vi "Signals.vi"() -> ()   [LabVIEW 2016]
uses:
  controls/Enum.ctl
  <vilib>/rvi/errors/niLvFpgaAdjustHostInterfaceError.vi
  SubVIs/ConvertToVoltsArray.vi
  controls/FPGAVIreferenceTypeDef.ctl
  <vilib>/rvi/interface/nirviReadWriteControl/nirviReadWriteControl.xnode
  FPGA Bitfiles/lbniAFMControlle_flexRio_controllerFPGA.lvbitx
  controls/FPGAVIreferenceTypeDefScanEngine.ctl
  FPGA Bitfiles/lbniAFMControlle_scanControl_controllerFPGAPX_N4i+37z1gG8.lvbitx
  Course Project/support/Message Queue/Message Queue.lvlib
  Course Project/support/User Event - Stop/User Event - Stop.lvlib
  NiFpgaLv.dll
panel:
  in  "channelConfiguration":enum32{"Signal"}(tab)
  in  "Signals":enum32{"Overview", "Selection"}(tab)
  in  "Analog inputs":T1={"Unit"={"Unit 1"="m", "Unit 2"="V", "Unit 3"="V", "Unit 4"="V", "Unit 5"="V", "Unit 6"="V", "Unit 7"="V", "Unit 8"="V"}, "Measurement"={"AI0 value"=0.0, "AI1 value"=0.0, "AI2 value"=0.0, "AI3 value"=-10.0, "AI4 value"=-10.0, "AI5 value"=-10.0, "AI6value"=-10.0, "AI7 value"=-10.0}, "Name"={"AI0 name"="Current", "AI1 name"="AI1", "AI2 name"="AI2", "AI3 name"="AI3", "AI4 name"="AI4", "AI5 name"="AI5", "AI6 name"="AI6", "AI7 name"="AI7"}, "Port"={"AI0"="AI0", "AI1"="AI1", "AI2"="AI2", "AI3"="AI3", "AI4"="AI4", "AI5"="AI5", "AI6"="AI6", "AI7"="AI7"}, "Calibration"={"Meas 1"=1.0, "Meas 2"=1.0, "Meas 3"=1.0, "Meas 4"=1.0, "Meas 5"=1.0, "Meas 6"=1.0, "Meas 7"=1.0, "Meas 8"=1.0}, "Offset"={"Unit 1"=0.0, "Unit 2"=0.0, "Unit 3"=0.0, "Unit 4"=0.0, "Unit 5"=0.0, "Unit 6"=0.0, "AI 106"=0.0, "Unit 8"=0.0}} {"Offset"."Unit 8" format="%#_3p"; "Offset"."AI 106" format="%#_3p"; "Offset"."Unit 6" format="%#_3p"; "Offset"."Unit 5" format="%#_3p"; "Offset"."Unit 4" format="%#_3p"; "Offset"."Unit 3" format="%#_3p"; "Offset"."Unit 2" format="%#_3p"; "Offset"."Unit 1" format="%#_3p"; "Calibration"."Meas 8" format="%#_3p"; "Calibration"."Meas 7" format="%#_3p"; "Calibration"."Meas 6" format="%#_3p"; "Calibration"."Meas 5" format="%#_3p"; "Calibration"."Meas 4" format="%#_3p"; "Calibration"."Meas 3" format="%#_3p"; "Calibration"."Meas 2" format="%#_3p"; "Calibration"."Meas 1" format="%#_3p"; "Measurement"."AI7 value" format="%#_4g"; "Measurement"."AI6value" format="%#_4g"; "Measurement"."AI5 value" format="%#_4p"; "Measurement"."AI4 value" format="%#_4p"; "Measurement"."AI3 value" format="%#_4p"; "Measurement"."AI2 value" format="%#_4p"; "Measurement"."AI1 value" format="%#_4p"; "Measurement"."AI0 value" format="%#_4p"}
  in  "Analog outputs":T2={"Unit"={"Unit 4"="V", "Unit 5"="V", "Unit 6"="V", "AI 106"="V", "Unit 8"="V"}, "Measurement"={"Meas 4"=0.0, "Meas 5"=0.0, "Meas 6"=0.0, "Meas 7"=0.0, "Meas 8"=0.0}, "Name"={"AO3 name"="AO3", "AO4 name"="Bias", "AO5 name"="DC Motor", "AO6 name"="AO6", "AO7 name"="AO7"}, "Port"={"A03"="AO3", "A04"="AO4", "A05"="AO5", "A06"="AO6", "A00"="AO7"}, "Calibration"={"Meas 4"=1.0, "Meas 5"=1.0, "Meas 6"=1.0, "Meas 7"=1.0, "Meas 8"=1.0}, "Offset"={"Unit 4"=0.0, "Unit 5"=0.0, "Unit 6"=0.0, "AI 106"=0.0, "Unit 8"=0.0}} {"Offset"."Unit 8" format="%#_3p"; "Offset"."AI 106" format="%#_3p"; "Offset"."Unit 6" format="%#_3p"; "Offset"."Unit 5" format="%#_3p"; "Offset"."Unit 4" format="%#_3p"; "Calibration"."Meas 8" format="%#_3p"; "Calibration"."Meas 7" format="%#_3p"; "Calibration"."Meas 6" format="%#_3p"; "Calibration"."Meas 5" format="%#_3p"; "Calibration"."Meas 4" format="%#_3p"; "Measurement"."Meas 8" format="%#_4p"; "Measurement"."Meas 7" format="%#_4p"; "Measurement"."Meas 6" format="%#_4p"; "Measurement"."Meas 5" format="%#_4p"; "Measurement"."Meas 4" format="%#_4p"}
  in  "XYZ":T3={"Unit"={"Unit 1"="m", "Unit 2"="m", "Unit 3"="m"}, "Measurement"={"Meas 1"=0.0, "Meas 2"=0.0, "Meas 3"=0.0}, "Name"={"AO0 name"="X", "AO1 name"="Y", "AO2 name"="Z"}, "Port"={"A00"="AO0", "A01"="AO1", "A02"="AO2"}, "Calibration"={"Meas 1"=1.0, "Meas 2"=1.0, "Meas 3"=1.0}, "Offset"={"Unit 1"=0.0, "Unit 2"=0.0, "Unit 3"=0.0}} {"Offset"."Unit 3" format="%#_3p"; "Offset"."Unit 2" format="%#_3p"; "Offset"."Unit 1" format="%#_3p"; "Calibration"."Meas 3" format="%#_3p"; "Calibration"."Meas 2" format="%#_3p"; "Calibration"."Meas 1" format="%#_3p"; "Measurement"."Meas 3" format="%#_4p"; "Measurement"."Meas 2" format="%#_4p"; "Measurement"."Meas 1" format="%#_4p"}
  in  "Save to config file":bool
  in  "Channels to save":i32[](listbox)=[0, 1, 2, 3, 4, 5, 6, 7]
  in  "Update Time":i32=500
  in  "SavingChoice":T4={"Units"=-1, "Saving"={"Fwd"=[0, 1, 3, 4, 5], "Bwd"=[0, 1]}, "x"=[]}
  in  "assignementChoice":enum32{"Selection", "Overview", "Assignment"}(radio)
  # "Ch"
  # "Name"
  # "Value"
  # "Unit"
  # "Offset"
  # "Cal"
  # "Select the channels to save.\nFor multiple selection, press ctrl + mouse."
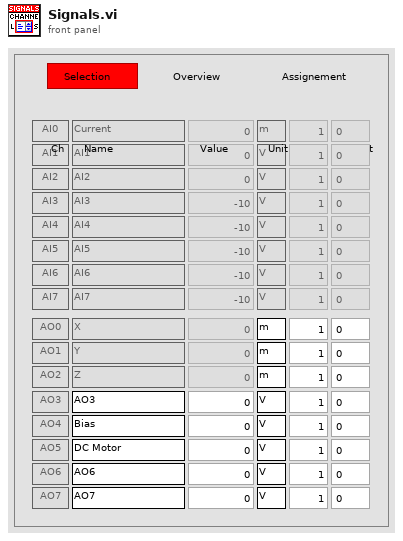
[diagram p1: front panel]
types:
  T1 = cluster{"Unit":cluster{"Unit 1":string, "Unit 2":string, "Unit 3":string, "Unit 4":string, "Unit 5":string, "Unit 6":string, "Unit 7":string, "Unit 8":string}, "Measurement":cluster{"AI0 value":dbl, "AI1 value":dbl, "AI2 value":dbl, "AI3 value":dbl, "AI4 value":dbl, "AI5 value":dbl, "AI6value":dbl, "AI7 value":dbl}, "Name":cluster{"AI0 name":string, "AI1 name":string, "AI2 name":string, "AI3 name":string, "AI4 name":string, "AI5 name":string, "AI6 name":string, "AI7 name":string}, "Port":cluster{"AI0":string, "AI1":string, "AI2":string, "AI3":string, "AI4":string, "AI5":string, "AI6":string, "AI7":string}, "Calibration":cluster{"Meas 1":dbl, "Meas 2":dbl, "Meas 3":dbl, "Meas 4":dbl, "Meas 5":dbl, "Meas 6":dbl, "Meas 7":dbl, "Meas 8":dbl}, "Offset":cluster{"Unit 1":dbl, "Unit 2":dbl, "Unit 3":dbl, "Unit 4":dbl, "Unit 5":dbl, "Unit 6":dbl, "AI 106":dbl, "Unit 8":dbl}}
  T2 = cluster{"Unit":cluster{"Unit 4":string, "Unit 5":string, "Unit 6":string, "AI 106":string, "Unit 8":string}, "Measurement":cluster{"Meas 4":dbl, "Meas 5":dbl, "Meas 6":dbl, "Meas 7":dbl, "Meas 8":dbl}, "Name":cluster{"AO3 name":string, "AO4 name":string, "AO5 name":string, "AO6 name":string, "AO7 name":string}, "Port":cluster{"A03":string, "A04":string, "A05":string, "A06":string, "A00":string}, "Calibration":cluster{"Meas 4":dbl, "Meas 5":dbl, "Meas 6":dbl, "Meas 7":dbl, "Meas 8":dbl}, "Offset":cluster{"Unit 4":dbl, "Unit 5":dbl, "Unit 6":dbl, "AI 106":dbl, "Unit 8":dbl}}
  T3 = cluster{"Unit":cluster{"Unit 1":string, "Unit 2":string, "Unit 3":string}, "Measurement":cluster{"Meas 1":dbl, "Meas 2":dbl, "Meas 3":dbl}, "Name":cluster{"AO0 name":string, "AO1 name":string, "AO2 name":string}, "Port":cluster{"A00":string, "A01":string, "A02":string}, "Calibration":cluster{"Meas 1":dbl, "Meas 2":dbl, "Meas 3":dbl}, "Offset":cluster{"Unit 1":dbl, "Unit 2":dbl, "Unit 3":dbl}}
  T4 = cluster{"Units":i32, "Saving":cluster{"Fwd":i32[], "Bwd":i32[]}, "x":i32[]}
  T5 = typedef "Enum.ctl" = enum16{"Init", "Read", "Write"}
  T6 = enum8{"Enabled", "Disabled", "Disabled and Grayed Out"}
  T7 = typedef "Message Queue.lvlib/All Message Queues.ctl" = cluster{"IU":refnum<queue>}
  T8 = typedef "FPGAVIreferenceTypeDef.ctl" = refnum<k20>
  T9 = typedef "FPGAVIreferenceTypeDefScanEngine.ctl" = refnum<k20>
  T10 = cluster{"Unit 1":string, "Unit 2":string, "Unit 3":string}
  T11 = cluster{"Meas 1":dbl, "Meas 2":dbl, "Meas 3":dbl}
  T12 = cluster{"Unit 1":dbl, "Unit 2":dbl, "Unit 3":dbl}
  T13 = cluster{"Unit 1":string, "Unit 2":string, "Unit 3":string, "Unit 4":string, "Unit 5":string, "Unit 6":string, "Unit 7":string, "Unit 8":string}
  T14 = cluster{"Unit 4":string, "Unit 5":string, "Unit 6":string, "AI 106":string, "Unit 8":string}
  T15 = cluster{"Unit 1":dbl, "Unit 2":dbl, "Unit 3":dbl, "Unit 4":dbl, "Unit 5":dbl, "Unit 6":dbl, "AI 106":dbl, "Unit 8":dbl}
  T16 = cluster{"Unit 4":dbl, "Unit 5":dbl, "Unit 6":dbl, "AI 106":dbl, "Unit 8":dbl}
  T17 = cluster{"Meas 1":dbl, "Meas 2":dbl, "Meas 3":dbl, "Meas 4":dbl, "Meas 5":dbl, "Meas 6":dbl, "Meas 7":dbl, "Meas 8":dbl}
  T18 = cluster{"Meas 4":dbl, "Meas 5":dbl, "Meas 6":dbl, "Meas 7":dbl, "Meas 8":dbl}
  T19 = cluster{"channelsToSaveOut":u8[], "Units":string[], "Saving":cluster{"Fwd":i32[], "Bwd":i32[]}, "x":i32[]}
  T20 = cluster{"Units":string[], "Offsets":dbl[], "Calibrations":dbl[]}
  T21 = cluster{"calibName":string[], "calibParameters":cluster{"Sensitivity":cluster{"Sens X":dbl, "Sens Y":dbl, "Sens Z":dbl}, "Range":cluster{"Range X":dbl, "Range Y":dbl, "Range Z":dbl}, "HV gain":cluster{"HV gain X":dbl, "HV gain Y":dbl, "HV gain Z":dbl}}[], "calibIndex":i32}
  T22 = cluster{"Sensitivity":cluster{"Sens X":dbl, "Sens Y":dbl, "Sens Z":dbl}, "Range":cluster{"Range X":dbl, "Range Y":dbl, "Range Z":dbl}, "HV gain":cluster{"HV gain X":dbl, "HV gain Y":dbl, "HV gain Z":dbl}}[]
  T23 = cluster{"Sensitivity":cluster{"Sens X":dbl, "Sens Y":dbl, "Sens Z":dbl}, "Range":cluster{"Range X":dbl, "Range Y":dbl, "Range Z":dbl}, "HV gain":cluster{"HV gain X":dbl, "HV gain Y":dbl, "HV gain Z":dbl}}
  T24 = cluster{"AI0 value":dbl, "AI1 value":dbl, "AI2 value":dbl, "AI3 value":dbl, "AI4 value":dbl, "AI5 value":dbl, "AI6value":dbl, "AI7 value":dbl}
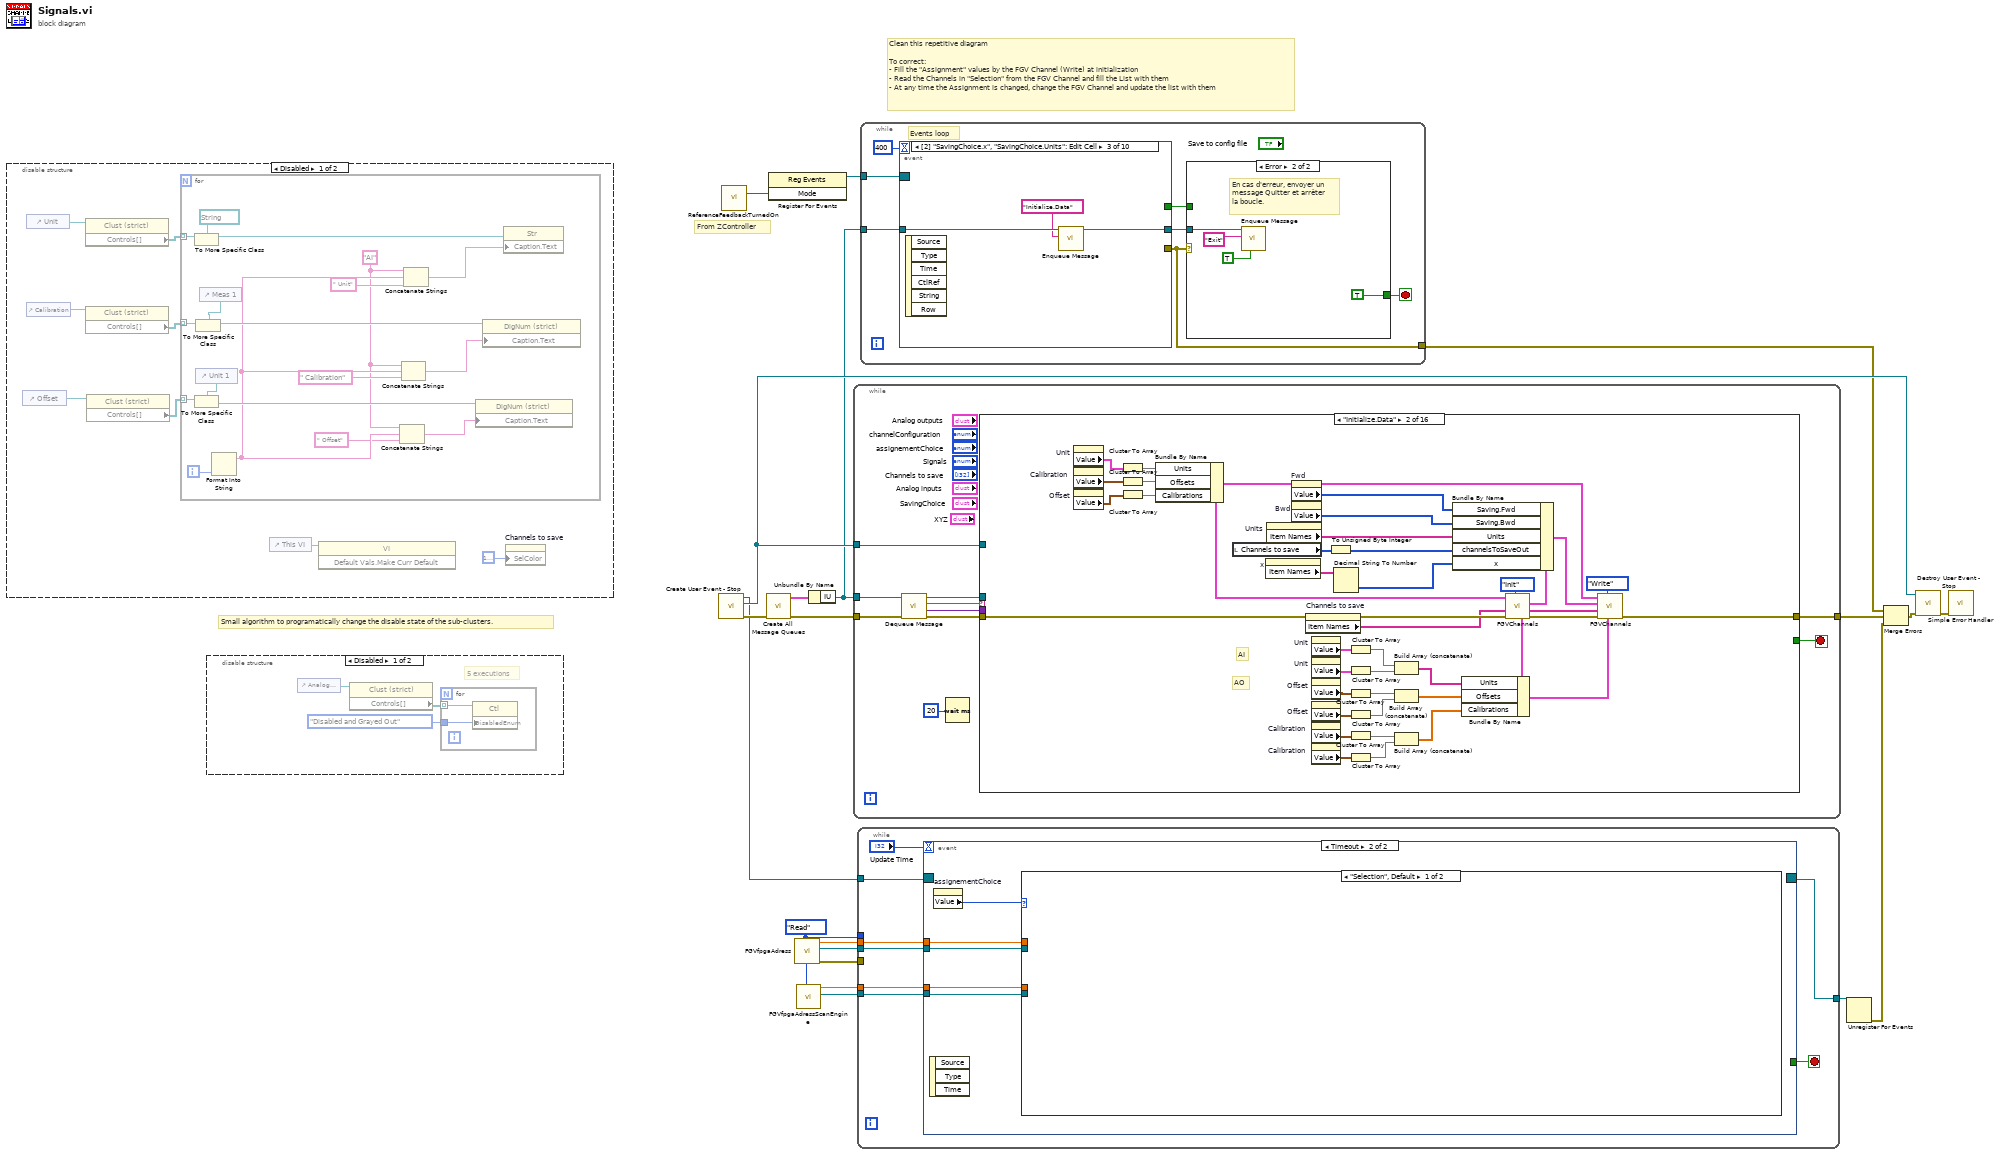
[diagram p0: block diagram]
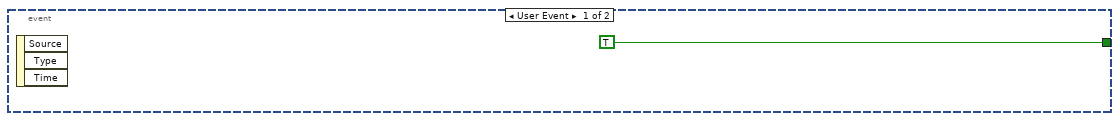
[diagram p2: hidden frame]
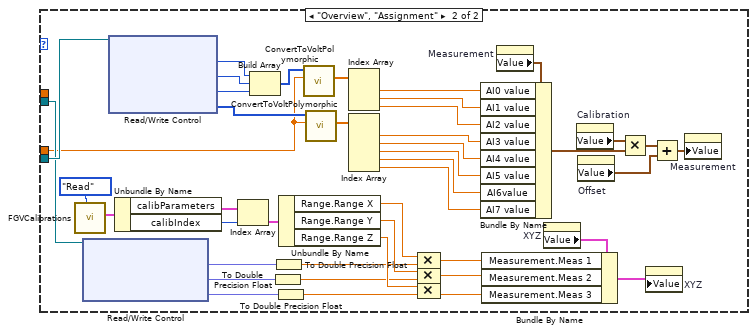
[diagram p3: hidden frame]
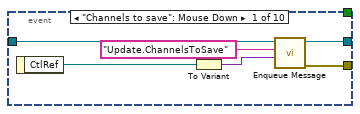
[diagram p5: hidden frame]
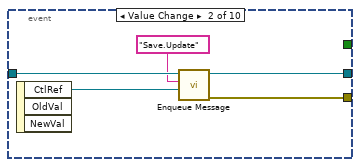
[diagram p6: hidden frame]
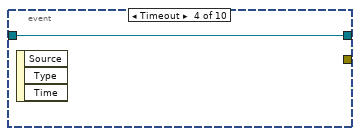
[diagram p7: hidden frame]
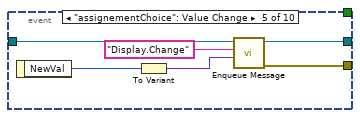
[diagram p8: hidden frame]
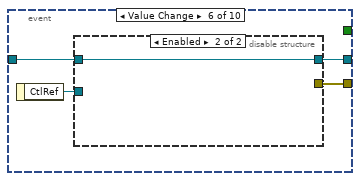
[diagram p9: hidden frame]
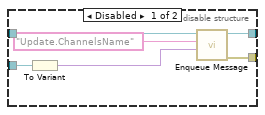
[diagram p10: hidden frame]
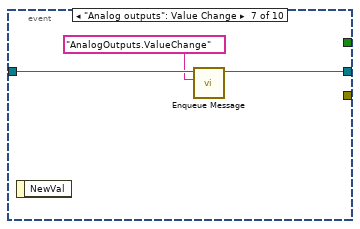
[diagram p11: hidden frame]
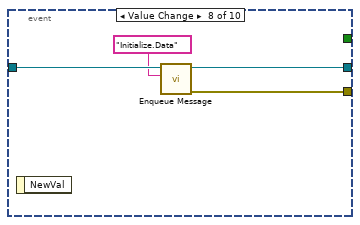
[diagram p12: hidden frame]
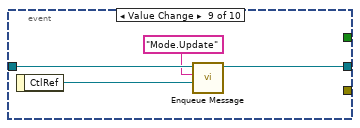
[diagram p13: hidden frame]
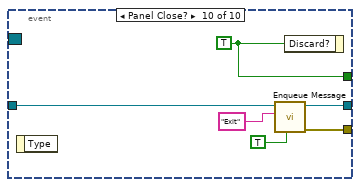
[diagram p14: hidden frame]
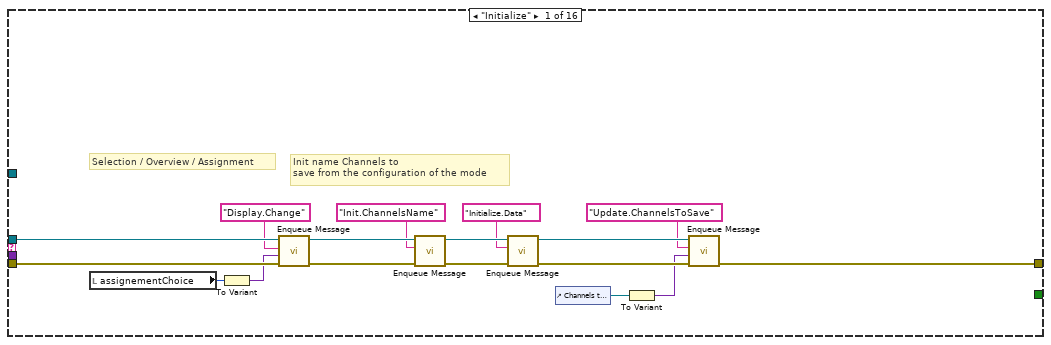
[diagram p15: hidden frame]
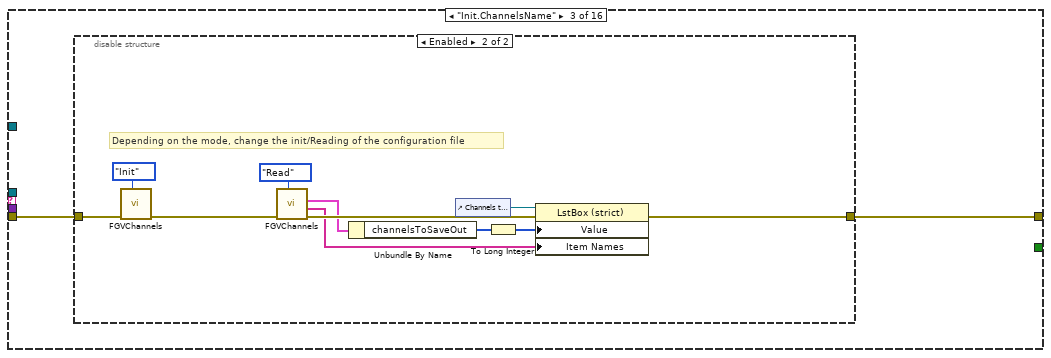
[diagram p16: hidden frame]
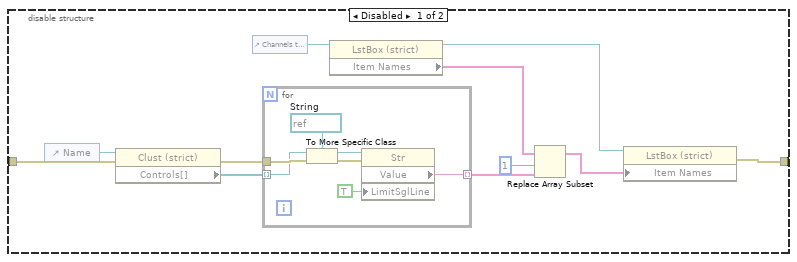
[diagram p17: hidden frame]
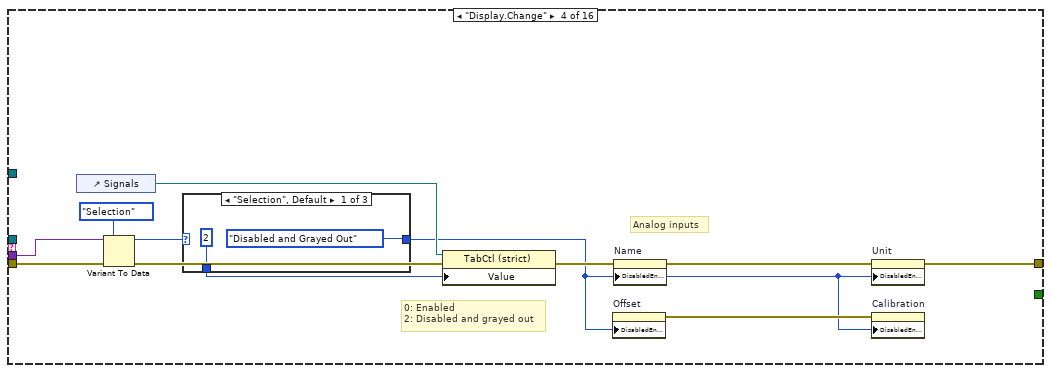
[diagram p18: hidden frame]
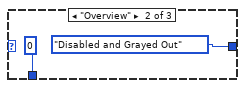
[diagram p19: hidden frame]
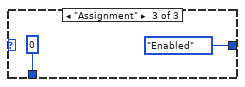
[diagram p20: hidden frame]
diagram:
  w6 = Enum."Read" ("Enum")
  # "Clean this repetitive diagram\n\nTo correct:\n- Fill the \"Assignment\" values by the FGV Channel (Write) at initialization\n- Read the Channels in \"Selection\" from the FGV Channel and fill the List with them\n- At any time the Assignment is changed, change the FGV Channel and update the list with them"
  # "From ZController"
  # "Small algorithm to programatically change the disable state of the sub-clusters."
  n1 = disable-structure shown="Disabled" {
    frame Disabled {
      n2 = control-ref of="Offset"() -> (w26:refnum<vi>)
      n3 = control-ref of="Unit"() -> (w28:refnum<vi>)
      n4 = control-ref of="Calibration"() -> (w27:refnum<vi>)
      n5 = property class="Clust (strict)"(reference=w28) -> ("Controls[]"=w25:refnum<vi>[])  [unwired: 1 in, 2 out]
      n6 = property class="Clust (strict)"(reference=w27) -> ("Controls[]"=w24:refnum<vi>[])  [unwired: 1 in, 2 out]
      n7 = property class="Clust (strict)"(reference=w26) -> ("Controls[]"=w23:refnum<vi>[])  [unwired: 1 in, 2 out]
      n8 = for {
        tunnel: w25 -> [w46] mode=indexing
        tunnel: w24 -> [w44] mode=indexing
        tunnel: w23 -> [w43] mode=indexing
        i -> [w39]
        w29 = "AI"
        n9 = To More Specific Class(target class=refnum<vi> refnum ("Unit 1"), reference=w46) -> (specific class reference=w40:refnum<vi>)  [unwired: 1 in, 1 out]
        n10 = control-ref of="Unit 1"() -> (w30:refnum<vi>)
        n11 = To More Specific Class(target class=w30, reference=w43) -> (specific class reference=w42:refnum<vi>)  [unwired: 1 in, 1 out]
        n12 = control-ref of="Meas 1"() -> (w31:refnum<vi>)
        n13 = To More Specific Class(target class=w31, reference=w44) -> (specific class reference=w41:refnum<vi>)  [unwired: 1 in, 1 out]
        n14 = Format Into String(w39) -> (resulting string=w38:string)  [unwired: 3 in, 1 out]
        n15 = Concatenate Strings(w29, w38, " Offset") -> (w32:string)
        n16 = Concatenate Strings(w29, w38, " Calibration") -> (w33:string)
        n17 = Concatenate Strings(w29, w38, " Unit") -> (w34:string)
        n18 = property class="DigNum (strict)"(reference=w42, "Caption.Text"=w32) -> ()  [unwired: 1 in, 2 out]
        n19 = property class="DigNum (strict)"(reference=w41, "Caption.Text"=w33) -> ()  [unwired: 1 in, 2 out]
        n20 = property class="Str"(reference=w40, "Caption.Text"=w34) -> ()  [unwired: 1 in, 2 out]
      }
      n21 = control-ref of="This VI"() -> (w22:refnum<vi>)
      n22 = invoke class="VI" method="Default Vals.Make Curr Default"(reference=w22) -> ()  [unwired: 2 in, 3 out]
      n23 = property on="Channels to save" class="LstBox (strict)"("SelColor"=u32 16777224) -> ()  [unwired: 2 in, 2 out]
    }
    frame Enabled {
    }
  }
  n24 = disable-structure shown="Disabled" {
    frame Disabled {
      # "5 executions"
      n25 = control-ref of="Analog inputs"() -> (w49:refnum<vi>)
      n26 = property class="Clust (strict)"(reference=w49) -> ("Controls[]"=w48:refnum<vi>[])  [unwired: 1 in, 2 out]
      n27 = for {
        tunnel: w48 -> [w51] mode=indexing
        tunnel: T6."Disabled and Grayed Out" ("Disabled") -> [w50]
        n28 = property class="Ctl"(reference=w51, "DisabledEnum"=w50) -> ()  [unwired: 1 in, 2 out]
      }
    }
    frame Enabled {
    }
  }
  n29 = call "Create User Event - Stop.vi"() -> ("sortie d'erreur"=w17:errorcluster, "Événement utilisateur - Arrêt"=w20:refnum<user-event>, "Refnum Enregistrement à l'événement Arrêt"=w10:refnum<event-registration>)  [unwired: 9 in]
  n30 = call "ReferenceFeedbackTurnedOn.vi"() -> ("Mode"=w1:refnum<vi>)  [unwired: 9 in, 2 out]
  n31 = call "Create All Message Queues.vi"("ErrorIn"=w17) -> ("ErrorOut"=w13:errorcluster, "MessageQueueOut"=w14:T7)  [unwired: 9 in]
  n32 = register-events(w1) -> (reference out=w2:refnum<event-registration>)  [unwired: 2 in, 1 out]
  n33 = call "FGVfpgaAdress.vi"("Enum"=w6) -> ("error out"=w12:errorcluster, "FPGA VI Reference Out"=w11:T8, "voltageRange(+/-)Out"=w3:dbl)  [unwired: 5 in, 3 out]
  n34 = call "FGVfpgaAdressScanEngine.vi"("Enum"=w6) -> ("FPGA.SEout"=w5:T9, "voltageRange(+/-)Out"=w4:dbl)  [unwired: 6 in, 3 out]
  n35 = Unbundle By Name(w14) -> ("IU"=w16:refnum<queue>)
  n36 = while {
    tunnel: w16 -> [w53]
    tunnel: w20 -> [w59]
    tunnel: w13 -> [w58]
    tunnel: [w60] -> w15
    stop <- w61 stop-if-true
    n37 = call "Dequeue Message.vi"("entrée d'erreur (pas d'erreur)"=w58, "File d'attente de messages"=w53) -> ("sortie d'erreur"=w57:errorcluster, "Données de message"=w55:variant, "Message"=w56:string, "File d'attente de message dup."=w54:refnum<queue>)  [unwired: 6 in]
    n38 = Wait (ms)(milliseconds to wait=u32 20) -> ()  [unwired: 1 out]
    n39 = case "Conditions des messages" shown="\"Initialize.Data\"" w56 {
      selector: w56 -> [_ _ _ _ _ _ _ _ _ _ _ _ _ _ _ w408]
      tunnel: w54 -> [w75 _ _ _ _ _ _ _ _ _ _ _ w386 w397 w404 _]
      tunnel: w57 -> [w74 w95 w119 w161 w186 w228 w255 w275 w331 w342 w366 w372 w374 w395 w400 _]
      tunnel: [w66 w116 w120 w153 w180 w194 w256 w288 w330 w338 w359 w372 w380 w394 w401 w406] -> w60
      tunnel: [_ _ _ _ _ _ _ _ _ _ _ _ _ _ TRUE _] -> w61
      tunnel: w55 -> [_ _ _ w160 w185 w227 _ _ _ _ w365 _ _ _ _ _]
      tunnel: w59 -> [_ _ _ _ _ _ _ _ _ _ _ _ _ _ w399 _]
      frame "Initialize" {
        # "Selection / Overview / Assignment"
        # "Init name Channels to \nsave from the configuration of the mode"
        n40 = local read "assignementChoice"() -> (w62:enum32{"Selection", "Overview", "Assignment"})
        n41 = To Variant(anything=w62) -> (Variant=w63:variant)
        n42 = call "Enqueue Message.vi"("error in"=w74, "Data"=w63, "Message"="Display.Change", "Queue"=w75) -> ("error out"=w71:errorcluster, "Queue dup."=w76:refnum<queue>)  [unwired: 6 in]
        n43 = call "Enqueue Message.vi"("error in"=w71, "Message"="Init.ChannelsName", "Queue"=w76) -> ("error out"=w70:errorcluster, "Queue dup."=w77:refnum<queue>)  [unwired: 7 in]
        n44 = call "Enqueue Message.vi"("error in"=w70, "Message"="Initialize.Data", "Queue"=w77) -> ("error out"=w67:errorcluster, "Queue dup."=w78:refnum<queue>)  [unwired: 7 in]
        n45 = control-ref of="Channels to save"() -> (w65:refnum<vi>)
        n46 = To Variant(anything=w65) -> (Variant=w64:variant)
        n47 = call "Enqueue Message.vi"("error in"=w67, "Data"=w64, "Message"="Update.ChannelsToSave", "Queue"=w78) -> ("error out"=w66:errorcluster)  [unwired: 6 in, 1 out]
      }
      frame "Initialize.Data" {
        # "AO"
        # "AI"
        n48 = property on="Unit" class="Clust (strict)"() -> ("Value"=w91:T10)  [unwired: 2 in, 2 out]
        n49 = property on="Calibration" class="Clust (strict)"() -> ("Value"=w89:T11)  [unwired: 2 in, 2 out]
        n50 = property on="Offset" class="Clust (strict)"() -> ("Value"=w87:T12)  [unwired: 2 in, 2 out]
        n51 = Cluster To Array(cluster=w91) -> (array=w90:string[])
        n52 = Cluster To Array(cluster=w89) -> (array=w88:dbl[])
        n53 = Cluster To Array(cluster=w87) -> (array=w86:dbl[])
        n54 = local read "Channels to save"() -> (w113:i32[])
        n55 = property on="x" class="LstBox (strict)"() -> ("Item Names"=w80:string[])  [unwired: 2 in, 2 out]
        n56 = property on="Units" class="LstBox (strict)"() -> ("Item Names"=w111:string[])  [unwired: 2 in, 2 out]
        n57 = property on="Fwd" class="LstBox (strict)"() -> ("Value"=w109:i32[])  [unwired: 2 in, 2 out]
        n58 = property on="Bwd" class="LstBox (strict)"() -> ("Value"=w110:i32[])  [unwired: 2 in, 2 out]
        n59 = property on="Channels to save" class="LstBox (strict)"(error in=w95) -> (error out=w118:errorcluster, "Item Names"=w92:string[])  [unwired: 1 in, 1 out]
        n60 = property on="Unit" class="Clust (strict)"() -> ("Value"=w85:T13)  [unwired: 2 in, 2 out]
        n61 = property on="Unit" class="Clust (strict)"() -> ("Value"=w84:T14)  [unwired: 2 in, 2 out]
        n62 = property on="Offset" class="Clust (strict)"() -> ("Value"=w104:T15)  [unwired: 2 in, 2 out]
        n63 = property on="Offset" class="Clust (strict)"() -> ("Value"=w102:T16)  [unwired: 2 in, 2 out]
        n64 = property on="Calibration" class="Clust (strict)"() -> ("Value"=w105:T17)  [unwired: 2 in, 2 out]
        n65 = property on="Calibration" class="Clust (strict)"() -> ("Value"=w103:T18)  [unwired: 2 in, 2 out]
        n66 = To Unsigned Byte Integer(number=w113) -> (unsigned 8bit integer=w112:u8[])
        n67 = Decimal String To Number(string=w80) -> (number=w79:i32[])  [unwired: 2 in, 1 out]
        n68 = Cluster To Array(cluster=w85) -> (array=w83:string[])
        n69 = Cluster To Array(cluster=w84) -> (array=w82:string[])
        n70 = Cluster To Array(cluster=w104) -> (array=w100:dbl[])
        n71 = Cluster To Array(cluster=w102) -> (array=w101:dbl[])
        n72 = Cluster To Array(cluster=w105) -> (array=w99:dbl[])
        n73 = Cluster To Array(cluster=w103) -> (array=w98:dbl[])
        n74 = Build Array (concatenate)(w83, w82) -> (w81:string[])
        n75 = Build Array (concatenate)(w100, w101) -> (w97:dbl[])
        n76 = Build Array (concatenate)(w99, w98) -> (w96:dbl[])
        n77 = call "FGVChannels.vi"("Enum"=Enum."Init") -> ("SavingChoiceOut"=w114:T19, "XYZ Units/Cal/Offset Out"=w93:T20, "Units/Cal/Offset Out"=w107:T20)  [unwired: 6 in, 2 out]
        n78 = Bundle By Name(cluster=w93, "Units"=w90, "Offsets"=w88, "Calibrations"=w86) -> (w94:T20)
        n79 = Bundle By Name(cluster=w114, "Saving.Fwd"=w109, "Saving.Bwd"=w110, "Units"=w111, "channelsToSaveOut"=w112, "x"=w79) -> (w108:T19)
        n80 = Bundle By Name(cluster=w107, "Units"=w81, "Offsets"=w97, "Calibrations"=w96) -> (w106:T20)
        n81 = call "FGVChannels.vi"("Units/Cal/Offset In"=w106, "Enum"=Enum."Write", "error in"=w118, "channelsNamesIn"=w92, "SavingChoiceIn"=w108, "XYZ Units/Cal/Offset In"=w94) -> ("error out"=w116:errorcluster)  [unwired: 1 in, 4 out]
      }
      frame "Init.ChannelsName" {
        n82 = disable-structure shown="Enabled" {
          disable-tunnel: [w125 w144] -> w120
          disable-tunnel: w119 -> [w121 w147]
          frame Disabled {
            n83 = control-ref of="Name"() -> (w122:refnum<vi>)
            n84 = property class="Clust (strict)"(reference=w122, error in=w121) -> (error out=w124:errorcluster, "Controls[]"=w123:refnum<vi>[])  [unwired: 1 out]
            n85 = control-ref of="Channels to save"() -> (w131:refnum<vi>)
            n86 = for {
              tunnel: w124 -> [w137]
              tunnel: [w134] -> w129 mode=indexing
              tunnel: w123 -> [w132] mode=indexing
              w138 = refnum<vi> refnum  # String
              n87 = To More Specific Class(target class=w138, reference=w132, error in=w137) -> (specific class reference=w136:refnum<vi>, error out=w135:errorcluster)
              n88 = property class="Str"(reference=w136, error in=w135, "LimitSglLine"=TRUE ("Limit To Single Line?")) -> ("Value"=w134:string)  [unwired: 2 out]
            }
            n89 = property class="LstBox (strict)"(reference=w131) -> (reference out=w127:refnum<vi>, "Item Names"=w130:string[])  [unwired: 1 in, 1 out]
            n90 = Replace Array Subset(array=w130, new element=w129, index=1) -> (w128:string[])
            n91 = property class="LstBox (strict)"(reference=w127, "Item Names"=w128) -> (error out=w125:errorcluster)  [unwired: 1 in, 1 out]
          }
          frame Enabled {
            # "Depending on the mode, change the init/Reading of the configuration file"
            n92 = call "FGVChannels.vi"("Enum"=Enum."Init", "error in"=w147) -> ("error out"=w146:errorcluster)  [unwired: 5 in, 4 out]
            n93 = call "FGVChannels.vi"("Enum"=Enum."Read", "error in"=w146) -> ("error out"=w145:errorcluster, "channelsNamesOut"=w142:string[], "SavingChoiceOut"=w141:T19)  [unwired: 5 in, 2 out]
            n94 = Unbundle By Name(w141) -> ("channelsToSaveOut"=w140:u8[])
            n95 = control-ref of="Channels to save"() -> (w143:refnum<vi>)
            n96 = To Long Integer(number=w140) -> (32bit integer=w139:i32[])
            n97 = property class="LstBox (strict)"(reference=w143, error in=w145, "Value"=w139, "Item Names"=w142) -> (error out=w144:errorcluster)  [unwired: 1 out]
          }
        }
      }
      frame "Display.Change" {
        # "Analog inputs"
        # "0: Enabled\n2: Disabled and grayed out"
        n98 = control-ref of="Signals"() -> (w157:refnum<vi>)
        n99 = Variant To Data(error in=w161, type=enum32{"Selection", "Overview", "Assignment"}."Selection" ("NewVal"), Variant=w160) -> (data=w158:enum32{"Selection", "Overview", "Assignment"}, error out=w156:errorcluster)
        n100 = case shown="\"Selection\", Default" w158 {
          tunnel: [2 0 0] -> w155
          tunnel: [T6."Disabled and Grayed Out" ("Disabled") T6."Disabled and Grayed Out" ("Disabled") T6."Enabled" ("Disabled")] -> w150
          frame "Selection", Default {
          }
          frame "Overview" {
          }
          frame "Assignment" {
          }
        }
        n101 = property class="TabCtl (strict)"(reference=w157, error in=w156, "Value"=w155) -> (error out=w152:errorcluster)  [unwired: 1 out]
        n102 = property on="Offset" class="Clust (strict)"("DisabledEnum"=w150) -> (error out=w154:errorcluster)  [unwired: 2 in, 1 out]
        n103 = property on="Name" class="Clust (strict)"(error in=w152, "DisabledEnum"=w150) -> (error out=w151:errorcluster)  [unwired: 1 in, 1 out]
        n104 = property on="Unit" class="Clust (strict)"(error in=w151, "DisabledEnum"=w150) -> (error out=w153:errorcluster)  [unwired: 1 in, 1 out]
        n105 = property on="Calibration" class="Clust (strict)"(error in=w154, "DisabledEnum"=w150) -> ()  [unwired: 1 in, 2 out]
      }
      frame "Update.ChannelsName" {
        w171 = refnum<vi> refnum  # Cluster
        n106 = Variant To Data(error in=w186, type=refnum<vi> refnum ("CtlRef"), Variant=w185) -> (data=w183:refnum<vi>, error out=w184:errorcluster)
        n107 = property class="Clust (strict)"(reference=w183, error in=w184) -> (error out=w181:errorcluster, "Controls[]"=w182:refnum<vi>[], "Owner"=w172:refnum<vi>)  [unwired: 1 out]
        n108 = To More Specific Class(target class=w171, reference=w172) -> (specific class reference=w170:refnum<vi>)  [unwired: 1 in, 1 out]
        n109 = property class="Clust"(reference=w170) -> ("Label.Text"=w169:string)  [unwired: 1 in, 2 out]
        n110 = Equal?(x=w169, y="Analog inputs") -> ()  [unwired: 1 out]
        n111 = control-ref of="Channels to save"() -> (w177:refnum<vi>)
        n112 = for {
          tunnel: w182 -> [w192] mode=indexing
          tunnel: w181 -> [w191]
          tunnel: [w188] -> w175 mode=indexing
          w193 = refnum<vi> refnum  # String
          n113 = To More Specific Class(target class=w193, reference=w192, error in=w191) -> (specific class reference=w190:refnum<vi>, error out=w189:errorcluster)
          n114 = property class="Str"(reference=w190, error in=w189, "LimitSglLine"=TRUE ("Limit To Single Line?")) -> ("Value"=w188:string)  [unwired: 2 out]
        }
        n115 = property class="LstBox (strict)"(reference=w177) -> (reference out=w173:refnum<vi>, "Item Names"=w176:string[])  [unwired: 1 in, 1 out]
        n116 = Replace Array Subset(array=w176, new element=w175, index=0) -> (w174:string[])
        n117 = property class="LstBox (strict)"(reference=w173, "Item Names"=w174) -> (error out=w180:errorcluster)  [unwired: 1 in, 1 out]
      }
      frame "Update.ChannelsToSave" {
        n118 = Variant To Data(error in=w228, type=refnum<vi> refnum ("CtlRef"), Variant=w227) -> (data=w223:refnum<vi>, error out=w224:errorcluster)
        n119 = property on="Fwd" class="LstBox (strict)"() -> ("Value"=w212:i32[])  [unwired: 2 in, 2 out]
        n120 = property on="Bwd" class="LstBox (strict)"() -> ("Value"=w215:i32[])  [unwired: 2 in, 2 out]
        n121 = property class="LstBox (strict)"(reference=w223, error in=w224) -> (error out=w198:errorcluster, "Value"=w201:i32[], "Item Names"=w200:string[])  [unwired: 1 out]
        n122 = Array Size(array=w201) -> (size(s)=w202:i32)
        n123 = for {
          N: w202 -> [_]
          tunnel: w201 -> [w237]
          shift-right: [w234] -> w205
          shift-left: w212 -> [w236]
          shift-right: [w234] -> w207
          shift-left: w215 -> [w235]
          tunnel: w200 -> [w233]
          tunnel: w201 -> [w232] mode=indexing
          tunnel: [w231] -> w199 mode=indexing
          i -> [w238]
          n124 = Index Array(array=w235, index=w238) -> (element=w239:i32)
          n125 = Index Array(array=w237, index=w238) -> (element=w241:i32)
          n126 = Index Array(array=w233, index=w232) -> (element=w231:string)
          n127 = Index Array(array=w236, index=w238) -> (element=w242:i32)
          n128 = Not Equal?(x=w239, y=w241) -> (x != y?=w243:bool)
          n129 = Not Equal?(x=w242, y=w241) -> (x != y?=w244:bool)
          n130 = Compound Arithmetic op=AND(w244, w243) -> (w240:bool)
          n131 = case shown="False" w240 {
            tunnel: w241 -> [_ w249]
            tunnel: w238 -> [_ w246]
            tunnel: w235 -> [w245 w248]
            tunnel: [w245 w247] -> w234
            frame False {
            }
            frame True {
              n132 = Insert Into Array(array=w248, index=w246, new element=w249) -> (w247:i32[])
            }
          }
        }
        n133 = To Unsigned Byte Integer(number=w201) -> (unsigned 8bit integer=w210:u8[])
        n134 = property on="Units" class="LstBox (strict)"() -> ("Item Names"=w196:string[])  [unwired: 2 in, 2 out]
        n135 = Array Size(array=w207) -> (size(s)=w208:i32)
        n136 = Array Size(array=w205) -> (size(s)=w211:i32)
        n137 = property on="x" class="LstBox (strict)"(error in=w198) -> (error out=w230:errorcluster, "Item Names"=w217:string[])  [unwired: 1 in, 1 out]
        n138 = Subtract(x=w211, y=w202) -> (x-y=w209:i32)
        n139 = Subtract(x=w208, y=w202) -> (x-y=w206:i32)
        n140 = Absolute Value(x=w209) -> (abs(x)=w204:i32)
        n141 = Absolute Value(x=w206) -> (abs(x)=w203:i32)
        n142 = Decimal String To Number(string=w217) -> (number=w216:i32[])  [unwired: 2 in, 1 out]
        n143 = Delete From Array(array=w205, length=w204, index=w202) -> (array with subset deleted=w213:i32[])  [unwired: 1 out]
        n144 = Delete From Array(array=w207, length=w203, index=w202) -> (array with subset deleted=w214:i32[])  [unwired: 1 out]
        n145 = property on="Fwd" class="LstBox (strict)"("Value"=w213) -> ()  [unwired: 2 in, 2 out]
        n146 = property on="Bwd" class="LstBox (strict)"("Value"=w214) -> ()  [unwired: 2 in, 2 out]
        n147 = call "FGVChannels.vi"("Enum"=Enum."Read", "error in"=w230) -> ("error out"=w229:errorcluster, "SavingChoiceOut"=w219:T19, "XYZ Units/Cal/Offset Out"=w221:T20, "Units/Cal/Offset Out"=w220:T20)  [unwired: 5 in, 1 out]
        n148 = Bundle By Name(cluster=w219, "Units"=w196, "channelsToSaveOut"=w210, "Saving.Fwd"=w213, "Saving.Bwd"=w214, "x"=w216) -> (w218:T19)
        n149 = call "FGVChannels.vi"("Units/Cal/Offset In"=w220, "Enum"=Enum."Write", "error in"=w229, "channelsNamesIn"=w199, "SavingChoiceIn"=w218, "XYZ Units/Cal/Offset In"=w221) -> ("error out"=w195:errorcluster)  [unwired: 1 in, 4 out]
        n150 = call "FGVImageArray.vi"("Enum"=Enum."Init", "error in"=w195) -> ("error out"=w194:errorcluster)  [unwired: 8 in, 1 out]
      }
      frame "Save.Update" {
        n151 = property on="Fwd" class="LstBox (strict)"() -> ("Value"=w253:i32[])  [unwired: 2 in, 2 out]
        n152 = property on="Bwd" class="LstBox (strict)"() -> ("Value"=w252:i32[])  [unwired: 2 in, 2 out]
        n153 = call "FGVChannels.vi"("Enum"=Enum."Read", "error in"=w255) -> ("error out"=w261:errorcluster, "channelsNamesOut"=w254:string[], "SavingChoiceOut"=w250:T19, "XYZ Units/Cal/Offset Out"=w258:T20, "Units/Cal/Offset Out"=w257:T20)  [unwired: 5 in]
        n154 = Bundle By Name(cluster=w250, "Saving.Fwd"=w253, "Saving.Bwd"=w252) -> (w251:T19)
        n155 = call "FGVChannels.vi"("Units/Cal/Offset In"=w257, "Enum"=Enum."Write", "error in"=w261, "channelsNamesIn"=w254, "SavingChoiceIn"=w251, "XYZ Units/Cal/Offset In"=w258) -> ("error out"=w256:errorcluster)  [unwired: 1 in, 4 out]
      }
      frame "SendToFGV.Parameters" {
        # "X, Y, Z"
        # "AnalogOutputs"
        # "AnalogInputs"
        n156 = control-ref of="Channels to save"() -> (w276:refnum<vi>)
        n157 = property class="LstBox (strict)" props=["Value", "Item Names"](reference=w276, error in=w275) -> (error out=w274:errorcluster, "Value"=w273:i32[])  [unwired: 2 out]
        n158 = Array Size(array=w273) -> (size(s)=w287:i32)
        n159 = control-ref of="Unit"() -> (w272:refnum<vi>)
        n160 = control-ref of="Calibration"() -> (w271:refnum<vi>)
        n161 = control-ref of="Offset"() -> (w270:refnum<vi>)
        n162 = control-ref of="Unit"() -> (w286:refnum<vi>)
        n163 = control-ref of="Calibration"() -> (w285:refnum<vi>)
        n164 = control-ref of="Offset"() -> (w284:refnum<vi>)
        n165 = for {
          N: w287 -> [_]
          tunnel: w273 -> [w317]
          tunnel: w286 -> [w315]
          tunnel: [w312] -> w281 mode=indexing
          tunnel: w285 -> [w311]
          tunnel: w284 -> [w310]
          tunnel: [w304] -> w280 mode=indexing
          tunnel: [w303] -> w279 mode=indexing
          i -> [w316]
          n166 = property class="Clust (strict)"(reference=w315) -> ("Value"=w314:T13)  [unwired: 1 in, 2 out]
          n167 = property class="Clust (strict)"(reference=w311) -> ("Value"=w309:T17)  [unwired: 1 in, 2 out]
          n168 = property class="Clust (strict)"(reference=w310) -> ("Value"=w308:T15)  [unwired: 1 in, 2 out]
          n169 = Index Array(array=w317, index=w316) -> (element=w305:i32)
          n170 = Cluster To Array(cluster=w308) -> (array=w306:dbl[])
          n171 = Cluster To Array(cluster=w314) -> (array=w313:string[])
          n172 = Cluster To Array(cluster=w309) -> (array=w307:dbl[])
          n173 = Index Array(array=w313, index=w305) -> (element=w312:string)
          n174 = Index Array(array=w306, index=w305) -> (element=w303:dbl)
          n175 = Index Array(array=w307, index=w305) -> (element=w304:dbl)
        }
        n176 = for {
          N: 3 -> [_]
          tunnel: w272 -> [w296]
          tunnel: w271 -> [w295]
          tunnel: w270 -> [w294]
          tunnel: [w293] -> w267 mode=indexing
          tunnel: [w292] -> w262 mode=indexing
          tunnel: [w291] -> w266 mode=indexing
          i -> [w290]
          n177 = property class="Clust (strict)"(reference=w296) -> ("Value"=w302:T14)  [unwired: 1 in, 2 out]
          n178 = property class="Clust (strict)"(reference=w295) -> ("Value"=w300:T18)  [unwired: 1 in, 2 out]
          n179 = property class="Clust (strict)"(reference=w294) -> ("Value"=w299:T16)  [unwired: 1 in, 2 out]
          n180 = Cluster To Array(cluster=w299) -> (array=w297:dbl[])
          n181 = Cluster To Array(cluster=w302) -> (array=w301:string[])
          n182 = Cluster To Array(cluster=w300) -> (array=w298:dbl[])
          n183 = Index Array(array=w301, index=w290) -> (element=w293:string)
          n184 = Index Array(array=w297, index=w290) -> (element=w291:dbl)
          n185 = Index Array(array=w298, index=w290) -> (element=w292:dbl)
        }
        n186 = call "FGVChannels.vi"("Enum"=Enum."Read", "error in"=w274) -> ("error out"=w278:errorcluster, "channelsNamesOut"=w263:string[], "SavingChoiceOut"=w264:T19, "XYZ Units/Cal/Offset Out"=w268:T20, "Units/Cal/Offset Out"=w282:T20)  [unwired: 5 in]
        n187 = Bundle By Name(cluster=w282, "Units"=w281, "Calibrations"=w280, "Offsets"=w279) -> (w277:T20)
        n188 = Bundle By Name(cluster=w268, "Units"=w267, "Calibrations"=w262, "Offsets"=w266) -> (w265:T20)
        n189 = call "FGVChannels.vi"("Units/Cal/Offset In"=w277, "Enum"=Enum."Write", "error in"=w278, "channelsNamesIn"=w263, "SavingChoiceIn"=w264, "XYZ Units/Cal/Offset In"=w265) -> ("error out"=w288:errorcluster)  [unwired: 1 in, 4 out]
      }
      frame "AnalogOutputs.ValueChange" {
        n190 = call "FGVfpgaAdressScanEngine.vi"("Enum"=Enum."Read", "error in"=w331) -> ("error out"=w321:errorcluster, "FPGA.SEout"=w320:T9, "voltageRange(+/-)Out"=w318:dbl)  [unwired: 5 in, 2 out]
        n191 = property on="Measurement" class="Clust (strict)"(error in=w321) -> (error out=w329:errorcluster, "Controls[]"=w328:refnum<vi>[])  [unwired: 1 in, 1 out]
        n192 = for {
          tunnel: w328 -> [w332] mode=indexing
          tunnel: [w334] -> w327 mode=indexing
          tunnel: refnum<vi> refnum ("Meas 1") -> [w333]
          n193 = To More Specific Class(target class=w333, reference=w332) -> (specific class reference=w335:refnum<vi>)  [unwired: 1 in, 1 out]
          n194 = property class="DigNum (strict)"(reference=w335) -> ("Value"=w334:dbl)  [unwired: 1 in, 2 out]
        }
        n195 = Multiply(x=32768.0, y=w327) -> (x*y=w325:dbl[])
        n196 = Divide(x=w325, y=w318) -> (x/y=w324:dbl[])
        n197 = To Word Integer(number=w324) -> (16bit integer=w319:i16[])
        n198 = xnode "Read/Write Control"("FPGA VI Reference In"=w320, "error in"=w329, "aio.o.outputs"=w319) -> ("error out"=w330:errorcluster)  [unwired: 1 out]
      }
      frame "Ext.AOUpdate" {
        n199 = call "FGVfpgaAdressScanEngine.vi"("Enum"=Enum."Read", "error in"=w342) -> ("error out"=w341:errorcluster, "FPGA.SEout"=w340:T9)  [unwired: 5 in, 3 out]
        n200 = xnode "Read/Write Control"("FPGA VI Reference In"=w340, "error in"=w341) -> ("error out"=w339:errorcluster, "aio.o.outputs"=w337:i16[])  [unwired: 1 out]
        n201 = call-poly "ConvertToVoltPolymorphic.vi"("Channels"=w337) -> ("Volts"=w336:dbl[])  [unwired: 10 in]
        n202 = Index Array(array=w336) -> (element #1=w346:dbl, element #2=w347:dbl, element #3=w348:dbl, element #4=w349:dbl)  [unwired: 4 in]
        n203 = property on="Measurement" class="Clust (strict)"(error in=w339) -> (error out=w338:errorcluster, "Value"=w344:T18)  [unwired: 1 in, 1 out]
        n204 = Bundle By Name(cluster=w344, "Meas 5"=w346, "Meas 6"=w347, "Meas 7"=w348, "Meas 8"=w349) -> (w345:T18)
        n205 = property on="Measurement" class="Clust (strict)"("Value"=w345) -> ()  [unwired: 2 in, 2 out]
      }
      frame "Int.AOUpdate" {
        # "+ Event to update the other VI Front Panel"
        n206 = Variant To Data(error in=w366, type=refnum<vi> refnum ("Meas 4"), Variant=w365) -> (data=w356:refnum<vi>, error out=w355:errorcluster)
        n207 = property class="DigNum (strict)"(reference=w356, error in=w355) -> (error out=w354:errorcluster, "Label.Text"=w351:string, "Value"=w352:dbl)  [unwired: 1 out]
        n208 = case shown="\"Meas 5\"" w351 {
          tunnel: [0 4 1 2 3] -> w350
          frame "Meas 5" {
          }
          frame Default {
          }
          frame "Meas 6" {
          }
          frame "Meas 7" {
          }
          frame "Meas 8" {
          }
        }
        n209 = call "FGVfpgaAdress.vi"("Enum"=Enum."Read", "error in"=w354) -> ("error out"=w363:errorcluster, "FPGA VI Reference Out"=w362:T8)  [unwired: 4 in, 4 out]
        n210 = xnode "Read/Write Control"("FPGA VI Reference In"=w362, "error in"=w363) -> ("FPGA VI Reference Out"=w361:T8, "error out"=w360:errorcluster, "aio.o.outputs"=w358:i16[])
        n211 = Replace Array Subset(array=w358, new element=w352, index=w350) -> (w357:i16[])
        n212 = xnode "Read/Write Control"("FPGA VI Reference In"=w361, "error in"=w360, "aio.o.outputs"=w357) -> ("error out"=w359:errorcluster)  [unwired: 1 out]
      }
      frame "Refresh Measurements" {
        # "Height\nError\nAO0\n...\nAO8"
      }
      frame "Assignment.NameChange" {
        n213 = call "Enqueue Message.vi"("error in"=w374, "Message"="Init.ChannelsName", "Queue"=w386) -> ("error out"=w373:errorcluster)  [unwired: 7 in, 1 out]
        n214 = property on="Name" class="Clust (strict)"(error in=w373) -> (error out=w384:errorcluster, "Controls[]"=w383:refnum<vi>[])  [unwired: 1 in, 1 out]
        n215 = for {
          tunnel: w383 -> [w391] mode=indexing
          tunnel: w384 -> [w393]
          tunnel: [w388] -> w375
          tunnel: [w387] -> w377 mode=indexing
          n216 = To More Specific Class(target class=refnum<vi> refnum ("AI2 name"), reference=w391, error in=w393) -> (specific class reference=w390:refnum<vi>, error out=w389:errorcluster)
          n217 = property class="Str"(reference=w390, error in=w389) -> (error out=w388:errorcluster, "Value"=w387:string)  [unwired: 1 out]
        }
        n218 = call "FGVChannels.vi"("Enum"=Enum."Read", "error in"=w375) -> ("error out"=w385:errorcluster, "SavingChoiceOut"=w378:T19, "XYZ Units/Cal/Offset Out"=w379:T20)  [unwired: 5 in, 2 out]
        n219 = call "FGVChannels.vi"("Enum"=Enum."Write", "error in"=w385, "channelsNamesIn"=w377, "SavingChoiceIn"=w378, "XYZ Units/Cal/Offset In"=w379) -> ("error out"=w380:errorcluster)  [unwired: 2 in, 4 out]
      }
      frame "Mode.Update" {
        n220 = call "Enqueue Message.vi"("error in"=w395, "Message"="Init.ChannelsName", "Queue"=w397) -> ("error out"=w394:errorcluster)  [unwired: 7 in, 1 out]
      }
      frame "Exit" {
        n221 = call "Fire User Event - Stop.vi"("Événement utilisateur - Arrêt"=w399) -> ("sortie d'erreur"=w398:errorcluster)  [unwired: 10 in]
        n222 = Release Queue(queue=w404, error in (no error)=w400) -> (error out=w402:errorcluster)  [unwired: 1 in, 2 out]
        n223 = Merge Errors(w398, w402) -> (w401:errorcluster)
      }
      frame Default {
        n224 = Format Into String(format string="The message\"%s\" received in the gestion loop is not valid" ("Texte de message d'erreur inconnu"), w408) -> (resulting string=w405:string)  [unwired: 2 in, 1 out]
        n225 = call <vilib>:"Error Cluster From Error Code.vi"("error message (\"\")"=w405, "error code (0)"=1 ("code d'erreur (0)")) -> ("error out"=w406:errorcluster)  [unwired: 7 in]
      }
    }
  }
  n226 = while {
    tunnel: w12 -> [_]
    tunnel: w11 -> [w412]
    tunnel: w10 -> [w417]
    tunnel: [w415] -> w7
    tunnel: w6 -> [_]
    tunnel: w5 -> [w410]
    tunnel: w4 -> [w411]
    tunnel: w3 -> [w413]
    stop <- w416 stop-if-true
    n227 = event shown="[1] Timeout" {
      selector: w417 -> [_ _]
      dyn-events: [_ _] -> w415
      timeout: "Update Time" -> [_ _]
      tunnel: [TRUE _] -> w416
      tunnel: w413 -> [_ w422]
      tunnel: w412 -> [_ w421]
      tunnel: w411 -> [_ w420]
      tunnel: w410 -> [_ w419]
      event User Event {
        n228 = event-data() -> ()  [unwired: 1 in, 3 out]
      }
      event Timeout {
        n229 = event-data() -> ()  [unwired: 1 in, 3 out]
        n230 = property on="assignementChoice" class="RadioBtnsControl (strict)"() -> ("Value"=w423:enum32{"Selection", "Overview", "Assignment"})  [unwired: 2 in, 2 out]
        n231 = case shown="\"Selection\", Default" w423 {
          tunnel: w421 -> [_ w449]
          tunnel: w419 -> [_ w454]
          tunnel: w420 -> [_ w431]
          tunnel: w422 -> [_ _]
          frame "Selection", Default {
          }
          frame "Overview", "Assignment" {
            n232 = call "FGVCalibrations.vi"("Enum"=Enum."Read") -> ("calibOut"=w448:T21)  [unwired: 9 in, 1 out]
            n233 = xnode "Read/Write Control"("FPGA VI Reference In"=w449) -> ("se.mot.s.origin.xOut"=w443:fxp<+/-,18,2>, "se.mot.s.origin.yOut"=w441:fxp<+/-,18,2>, "fb.o.height"=w439:fxp<+/-,31,4>)  [unwired: 1 in, 2 out]
            n234 = xnode "Read/Write Control"("FPGA VI Reference In"=w454) -> ("aio.s.slowVertical"=w463:i16, "aio.s.slowHoriz"=w462:i16, "aio.s.sum"=w461:i16, "aio.o.inputs"=w432:i16[])  [unwired: 1 in, 2 out]
            n235 = Unbundle By Name(w448) -> ("calibParameters"=w447:T22, "calibIndex"=w445:i32)
            n236 = Index Array(array=w447, index=w445) -> (element=w446:T23)
            n237 = Build Array(w463, w462, w461) -> (w451:i16[])
            n238 = To Double Precision Float(number=w441) -> (double precision float=w433:dbl)
            n239 = To Double Precision Float(number=w443) -> (double precision float=w434:dbl)
            n240 = To Double Precision Float(number=w439) -> (double precision float=w438:dbl)
            n241 = Unbundle By Name(w446) -> ("Range.Range X"=w444:dbl, "Range.Range Y"=w442:dbl, "Range.Range Z"=w440:dbl)
            n242 = call-poly "ConvertToVoltPolymorphic.vi"("Voltage Range"=w431, "Channels"=w451) -> ("Volts"=w450:dbl[])  [unwired: 9 in]
            n243 = call-poly "ConvertToVoltPolymorphic.vi"("Voltage Range"=w431, "Channels"=w432) -> ("Volts"=w430:dbl[])  [unwired: 9 in]
            n244 = Index Array(array=w450) -> (element #1=w460:dbl, element #2=w459:dbl, element #3=w458:dbl)  [unwired: 3 in]
            n245 = Index Array(array=w430) -> (element #1=w429:dbl, element #2=w428:dbl, element #3=w427:dbl, element #4=w426:dbl, element #5=w425:dbl)  [unwired: 5 in]
            n246 = Compound Arithmetic op=MULTIPLY(w444, w434) -> (w437:dbl)
            n247 = Compound Arithmetic op=MULTIPLY(w442, w433) -> (w436:dbl)
            n248 = Compound Arithmetic op=MULTIPLY(w440, w438) -> (w435:dbl)
            n249 = property on="Measurement" class="Clust (strict)"() -> ("Value"=w464:T24)  [unwired: 2 in, 2 out]
            n250 = Bundle By Name(cluster=w464, "AI0 value"=w460, "AI1 value"=w459, "AI2 value"=w458, "AI3 value"=w429, "AI4 value"=w428, "AI5 value"=w427, "AI6value"=w426, "AI7 value"=w425) -> (w453:T24)
            n251 = property on="XYZ" class="Clust (strict)"() -> ("Value"=w466:T3)  [unwired: 2 in, 2 out]
            n252 = Bundle By Name(cluster=w466, "Measurement.Meas 1"=w437, "Measurement.Meas 2"=w436, "Measurement.Meas 3"=w435) -> (w465:T3)
            n253 = property on="Calibration" class="Clust (strict)"() -> ("Value"=w452:T17)  [unwired: 2 in, 2 out]
            n254 = property on="Offset" class="Clust (strict)"() -> ("Value"=w456:T15)  [unwired: 2 in, 2 out]
            n255 = Multiply(x=w452, y=w453) -> (x*y=w457:cluster{dbl, dbl, dbl, dbl, dbl, dbl, dbl, dbl})
            n256 = property on="XYZ" class="Clust (strict)"("Value"=w465) -> ()  [unwired: 2 in, 2 out]
            n257 = Add(x=w457, y=w456) -> (x+y=w455:cluster{dbl, dbl, dbl, dbl, dbl, dbl, dbl, dbl})
            n258 = property on="Measurement" class="Clust (strict)"("Value"=w455) -> ()  [unwired: 2 in, 2 out]
          }
        }
      }
    }
  }
  n259 = while {
    tunnel: w16 -> [w473]
    tunnel: [w469] -> w9
    tunnel: w2 -> [w467]
    stop <- w471 stop-if-true
    # "Events loop"
    n260 = event shown="[2] \"SavingChoice.x\", \"SavingChoice.Units\": Edit Cell" {
      selector: w467 -> [_ _ _ _ _ _ _ _ _ _]
      dyn-events: _ -> [_ _ _ _ _ _ _ _ _ _]
      timeout: 400 -> [_ _ _ _ _ _ _ _ _ _]
      tunnel: [_ _ _ _ _ _ _ _ _ w527] -> w472
      tunnel: w473 -> [w484 w489 w492 w493 w497 w503 w513 w517 w521 w526]
      tunnel: [w482 w485 _ _ w495 w501 _ w514 _ w525] -> w469
      tunnel: [w483 w486 w490 w493 w496 w502 w512 w515 w520 w524] -> w470
      event "Channels to save": Mouse Down {
        n261 = event-data() -> ("CtlRef"=w480:refnum<vi>)  [unwired: 1 in]
        n262 = To Variant(anything=w480) -> (Variant=w479:variant)
        n263 = call "Enqueue Message.vi"("Data"=w479, "Message"="Update.ChannelsToSave", "Queue"=w484) -> ("error out"=w482:errorcluster, "Queue dup."=w483:refnum<queue>)  [unwired: 7 in]
      }
      event "SavingChoice.Saving.Fwd", "SavingChoice.Saving.Bwd": Value Change {
        n264 = event-data() -> ("CtlRef"=w487:refnum<vi>)  [unwired: 1 in, 2 out]
        n265 = call "Enqueue Message.vi"("Data"=w487, "Message"="Save.Update", "Queue"=w489) -> ("error out"=w485:errorcluster, "Queue dup."=w486:refnum<queue>)  [unwired: 7 in]
      }
      event "SavingChoice.x", "SavingChoice.Units": Edit Cell {
        n266 = event-data() -> ()  [unwired: 1 in, 6 out]
        n267 = call "Enqueue Message.vi"("Message"="Initialize.Data", "Queue"=w492) -> ("Queue dup."=w490:refnum<queue>)  [unwired: 8 in, 1 out]
      }
      event Timeout {
        n268 = event-data() -> ()  [unwired: 1 in, 3 out]
      }
      event "assignementChoice": Value Change {
        n269 = event-data() -> ("NewVal"=w499:enum32{"Selection", "Overview", "Assignment"})  [unwired: 1 in]
        n270 = To Variant(anything=w499) -> (Variant=w494:variant)
        n271 = call "Enqueue Message.vi"("Data"=w494, "Message"="Display.Change", "Queue"=w497) -> ("error out"=w495:errorcluster, "Queue dup."=w496:refnum<queue>)  [unwired: 7 in]
      }
      event "Analog inputs.Name": Value Change {
        n272 = event-data() -> ("CtlRef"=w500:refnum<vi>)  [unwired: 1 in]
        n273 = disable-structure shown="Enabled" {
          disable-tunnel: w503 -> [w509 w510]
          disable-tunnel: [w508 w510] -> w502
          disable-tunnel: [w507 _] -> w501
          disable-tunnel: w500 -> [w505 _]
          frame Disabled {
            n274 = To Variant(anything=w505) -> (Variant=w504:variant)
            n275 = call "Enqueue Message.vi"("Data"=w504, "Message"="Update.ChannelsName", "Queue"=w509) -> ("error out"=w507:errorcluster, "Queue dup."=w508:refnum<queue>)  [unwired: 7 in]
          }
          frame Enabled {
          }
        }
      }
      event "Analog outputs": Value Change {
        n276 = event-data() -> ()  [unwired: 1 in, 1 out]
        n277 = call "Enqueue Message.vi"("Message"="AnalogOutputs.ValueChange", "Queue"=w513) -> ("Queue dup."=w512:refnum<queue>)  [unwired: 8 in, 1 out]
      }
      event "Analog inputs.Unit", "Analog inputs.Calibration", "Analog inputs.Offset", "Analog outputs.Unit", "Analog outputs.Calibration", "Analog outputs.Offset": Value Change {
        n278 = event-data() -> ()  [unwired: 1 in, 1 out]
        n279 = call "Enqueue Message.vi"("Message"="Initialize.Data", "Queue"=w517) -> ("error out"=w514:errorcluster, "Queue dup."=w515:refnum<queue>)  [unwired: 8 in]
      }
      event Value Change {
        n280 = event-data() -> ("CtlRef"=w518:refnum<vi>)  [unwired: 1 in]
        n281 = call "Enqueue Message.vi"("Data"=w518, "Message"="Mode.Update", "Queue"=w521) -> ("Queue dup."=w520:refnum<queue>)  [unwired: 7 in, 1 out]
      }
      event Panel Close? {
        w527 = TRUE ("Rejeter ?")
        n282 = event-data() -> ()  [unwired: 1 in, 1 out]
        n283 = call "Enqueue Message.vi"("Prioritary message"=TRUE ("Message prioritaire ? (F)"), "Message"="Exit", "Queue"=w526) -> ("error out"=w525:errorcluster, "Queue dup."=w524:refnum<queue>)  [unwired: 7 in]
        n284 = event-data ("Event Filter Node")("Discard?"=w527) -> ()  [unwired: 1 in, 1 out]
      }
    }
    n285 = case shown="Error" w469 {
      tunnel: [w474 TRUE ("Rejeter ?")] -> w471
      tunnel: w472 -> [w474 _]
      tunnel: w470 -> [_ w477]
      frame No Error {
      }
      frame Error {
        # "En cas d'erreur, envoyer un message Quitter et arrêter la boucle."
        n286 = call "Enqueue Message.vi"("Prioritary message"=TRUE ("Message prioritaire ? (F)"), "Message"="Exit", "Queue"=w477) -> ()  [unwired: 7 in, 2 out]
      }
    }
  }
  n287 = Unregister For Events(event registration refnum=w7) -> (error out=w8:errorcluster)  [unwired: 1 in]
  n288 = Merge Errors(w9, w15, w8) -> (w19:errorcluster)
  n289 = call "Destroy User Event - Stop.vi"("entrée d'erreur (pas d'erreur)"=w19, "Événement utilisateur - Arrêt"=w20) -> ("sortie d'erreur"=w18:errorcluster)  [unwired: 9 in]
  n290 = call <vilib>:"Simple Error Handler.vi"("error in (no error)"=w18) -> ()  [unwired: 4 in, 5 out]
